vi "Write Plot config.vi"(8 "error in (no error)":errorcluster, 10 "Cluster":T1={"plots"=[], "X-axis"={"Name Label.Text"="", "Style"=0, "Tick Colors:Minor Tick Color"=0, "Tick Colors:Tick Color"=0, "Marker Colors:Text Color"=0, "Grid Colors:Major Color"=0, "Grid Colors:Minor Color"=0, "Mapping Mode"=0, "Flipped"=FALSE, "Name Label.Visible"=FALSE, "Name Label.Text Colors:Text Color"=0, "Scale Fit"=0, "Editable"=FALSE, "Range:Maximum"=0.0, "Range:Minimum"=0.0, "Offset and Multiplier:Multiplier"=0.0, "Offset and Multiplier:Offset"=0.0, "Name Label.Font:Size"=0, "Marker.Font:Size"=0, "Uniform Marker Spacing?"=TRUE, "Format String"=""}, "Y-axes"=[], "General"={"Title"="", "Time to Plot"=1800.0, "Title.Visible"=FALSE, "Sidebar.Visible"=FALSE, "Plot Area:Colors:BG Color"=0}} {"General"."Time to Plot" format="%<%M:%S>t"}, 11 "BlueSinglePlotConfig in":refnum<class "BlueSinglePlotConfig.lvclass">) -> (0 "error out":errorcluster, 3 "BlueSinglePlotConfig out":refnum<class "BlueSinglePlotConfig.lvclass">)   [LabVIEW 2021, in "BluePlot.lvlib" / "BlueSinglePlotConfig.lvclass"]
uses:
  BlueSinglePlotConfig.lvclass
  BlueSinglePlotConfig.lvclass/BlueSinglePlotConfig.ctl
  TypeDefs/plot attributes V2.ctl
  BluePlot.lvlib
  TypeDefs/plot properties V2.ctl
  TypeDefs/Plot scale axis properties.ctl
  TypeDefs/Plot general properties.ctl
  TypeDefs/plot load data V2.ctl
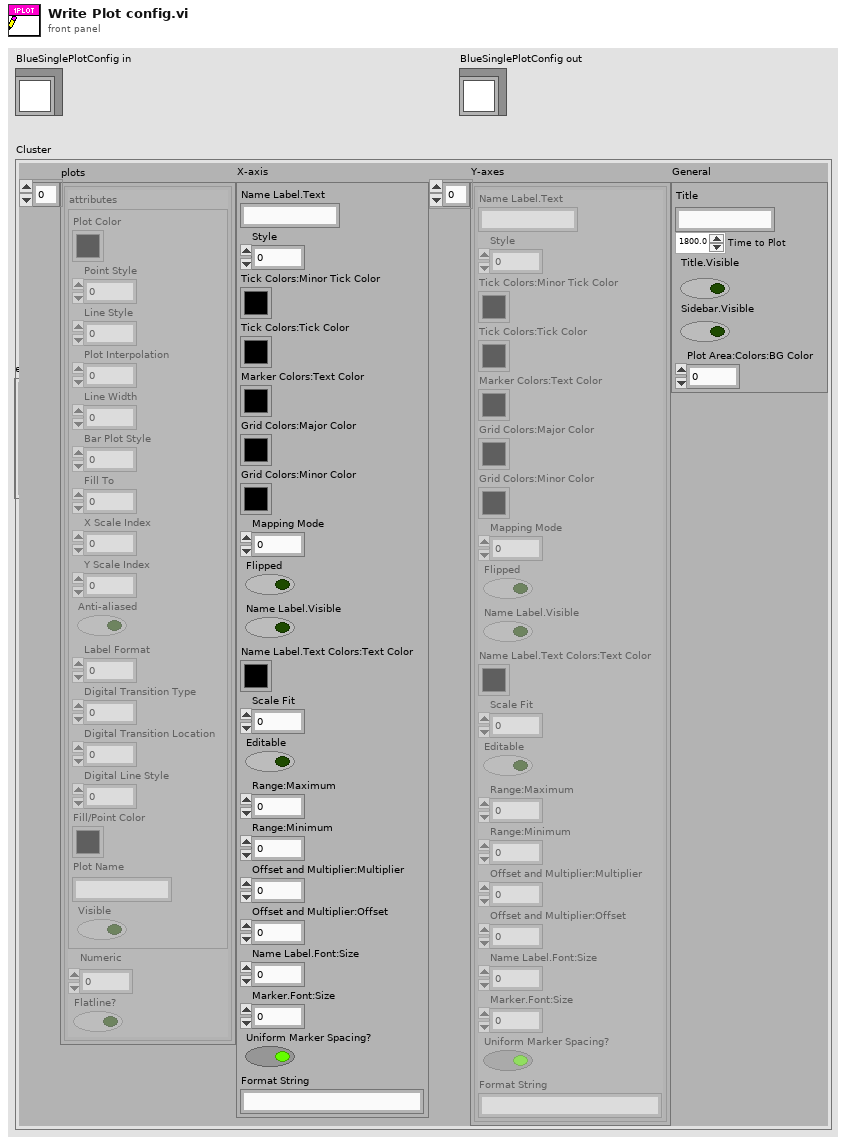
[diagram p1: front panel]
types:
  T1 = typedef "BluePlot.lvlib/plot load data V2.ctl" = cluster{"plots":T2[], "X-axis":T4, "Y-axes":T4[], "General":T5}
  T2 = typedef "BluePlot.lvlib/plot properties V2.ctl" = cluster{"attributes":T3, "Numeric":dbl, "Flatline?":bool}
  T3 = typedef "BluePlot.lvlib/plot attributes V2.ctl" = cluster{"Plot Color":u32, "Point Style":u8, "Line Style":u8, "Plot Interpolation":u8, "Line Width":u8, "Bar Plot Style":u8, "Fill To":i16, "X Scale Index":u32, "Y Scale Index":u32, "Anti-aliased":bool, "Label Format":u8, "Digital Transition Type":u8, "Digital Transition Location":u8, "Digital Line Style":u8, "Fill/Point Color":u32, "Plot Name":string, "Visible":bool}
  T4 = typedef "BluePlot.lvlib/Plot scale axis properties.ctl" = cluster{"Name Label.Text":string, "Style":u8, "Tick Colors:Minor Tick Color":u32, "Tick Colors:Tick Color":u32, "Marker Colors:Text Color":u32, "Grid Colors:Major Color":u32, "Grid Colors:Minor Color":u32, "Mapping Mode":u8, "Flipped":bool, "Name Label.Visible":bool, "Name Label.Text Colors:Text Color":u32, "Scale Fit":u8, "Editable":bool, "Range:Maximum":dbl, "Range:Minimum":dbl, "Offset and Multiplier:Multiplier":dbl, "Offset and Multiplier:Offset":dbl, "Name Label.Font:Size":u32, "Marker.Font:Size":u32, "Uniform Marker Spacing?":bool, "Format String":string}
  T5 = typedef "BluePlot.lvlib/Plot general properties.ctl" = cluster{"Title":string, "Time to Plot":dbl, "Title.Visible":bool, "Sidebar.Visible":bool, "Plot Area:Colors:BG Color":u32}
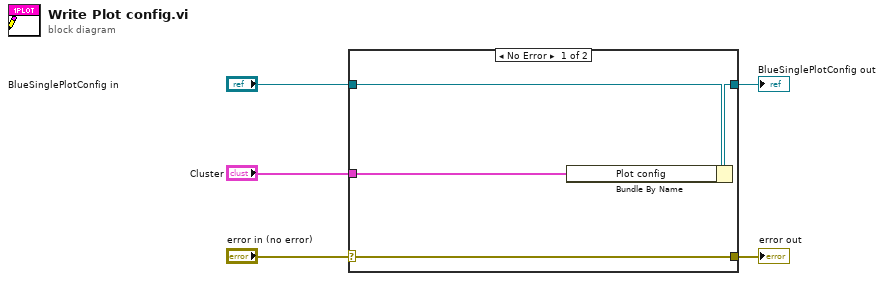
[diagram p0: block diagram]
diagram:
  n1 = case shown="No Error" "error in (no error)" {
    selector: "error in (no error)" -> [w9 w10]
    tunnel: [w9 w10] -> w4
    tunnel: [w7 w11] -> w2
    tunnel: "BlueSinglePlotConfig in" -> [w8 w11]
    tunnel: "Cluster" -> [w6 _]
    frame No Error {
      n2 = Bundle By Name(cluster=w8, "Plot config"=w6) -> (w7:refnum<class "BlueSinglePlotConfig.lvclass">)
    }
    frame Error {
    }
  }
  "error out" <- w4
  "BlueSinglePlotConfig out" <- w2
